vi "AlliGator Load Single Gate Image from SS2 mat File.vi"(6 "Action":T1, 8 "error in (no error)":errorcluster, 10 "File Info":variant, 11 "Gate Index":i32) -> (0 "error out":errorcluster, 1 "Data 2":sgl[][](array[numeric]), 3 "Data 1":sgl[][](array[numeric]))   [LabVIEW 2021, in "AlliGator Files.lvlib"]
doc: "Loads single gate image (or dual-channel images) from HDF5 FLI dataset file (v0.6b)."
uses:
  AlliGator Files.lvlib
  HDF5/AlliGator FLI Image Stack Action.ctl
  AlliGator SS2 mat FLI File Loading Information.ctl
  <vilib>/addons/h5labview2/file/H5F.lvlib
  GUI/AlliGator GUI.lvlib
  <vilib>/ErrorRing/Error Ring.xnode
  <vilib>/Utility/error.llb/Error Cluster From Error Code.vi
  <vilib>/addons/h5labview2/base/H5Equery.vi
  <vilib>/addons/h5labview2/base/lib_path.vi
  <vilib>/addons/h5labview2/dataset/H5Dread.llb/H5Dread.xnode
  HDF5/AlliGator HDF5.lvlib
panel:
  # "see the AlliGator License on the block diagram (Ctrl+E or Window:Show Block Diagram)"
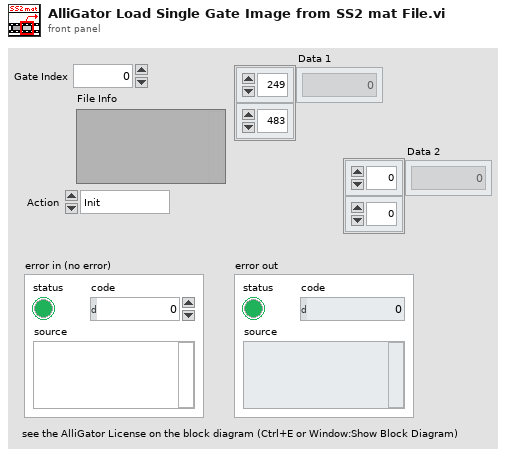
[diagram p1: front panel]
types:
  T1 = typedef "AlliGator HDF5.lvlib/AlliGator FLI Image Stack Action.ctl" = enum16{"Init", "Get Image", "Close"}
  T2 = typedef "AlliGator Files.lvlib/AlliGator SS2 mat FLI File Loading Information.ctl" = cluster{"mat File Path":path, "# Datasets":i32, "# Gates/Dataset":i32}
  T3 = typedef "hid_t.ctl" = i64
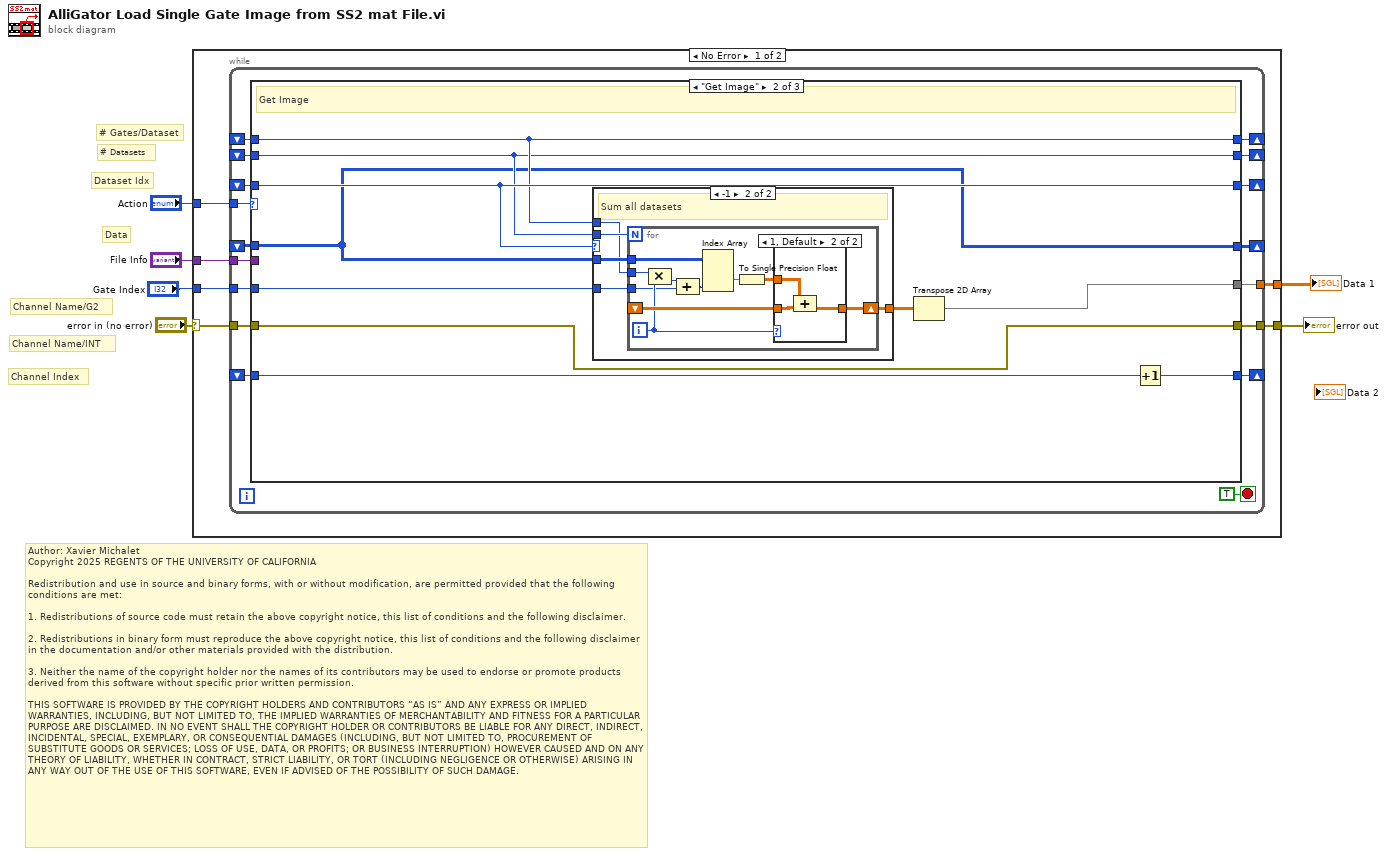
[diagram p0: block diagram]
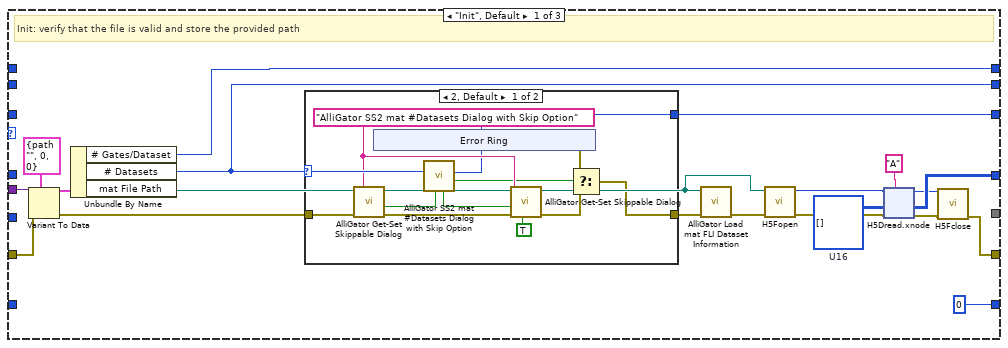
[diagram p2: hidden frame]
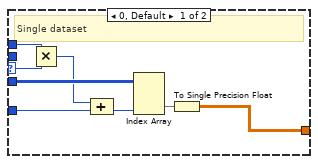
[diagram p4: hidden frame]
diagram:
  # "# Gates/Dataset"
  # "# Datasets"
  # "Dataset Idx"
  # "Data"
  # "Author: Xavier Michalet\nCopyright 2025 REGENTS OF THE UNIVERSITY OF CALIFORNIA\n\nRedistribution and use in source and binary forms, with or without modification, are permitted provided that the following conditions are met:\n\n1. Redistributions of source code must retain the above copyright notice, this list of conditions and the following disclaimer.\n\n2. Redistributions in binary form must reproduce the above copyright notice, this list of conditions and the following disclaimer in the documentation and/or other materials provided with the distribution.\n\n3. Neither the name of the copyright holder nor the names of its contributors may be used to endorse or promote products derived from this software without specific prior written permission.\n\nTHIS SOFTWARE IS PROVIDED BY THE COPYRIGHT HOLDERS AND CONTRIBUTORS “AS IS” AND ANY EXPRESS OR IMPLIED WARRANTIES, INCLUDING, BUT NOT LIMITED TO, THE IMPLIED WARRANTIES OF MERCHANTABILITY AND FITNESS FOR A PARTICULAR PURPOSE ARE DISCLAIMED. IN NO EVENT SHALL THE COPYRIGHT HOLDER OR CONTRIBUTORS BE LIABLE FOR ANY DIRECT, INDIRECT, INCIDENTAL, SPECIAL, EXEMPLARY, OR CONSEQUENTIAL DAMAGES (INCLUDING, BUT NOT LIMITED TO, PROCUREMENT OF SUBSTITUTE GOODS OR SERVICES; LOSS OF USE, DATA, OR PROFITS; OR BUSINESS INTERRUPTION) HOWEVER CAUSED AND ON ANY THEORY OF LIABILITY, WHETHER IN CONTRACT, STRICT LIABILITY, OR TORT (INCLUDING NEGLIGENCE OR OTHERWISE) ARISING IN ANY WAY OUT OF THE USE OF THIS SOFTWARE, EVEN IF ADVISED OF THE POSSIBILITY OF SUCH DAMAGE."
  # "Channel Index"
  # "Channel Name/INT"
  # "Channel Name/G2"
  n1 = case shown="No Error" "error in (no error)" {
    selector: "error in (no error)" -> [w11 w123]
    tunnel: [w10 w123] -> w5
    tunnel: "Action" -> [w12 _]
    tunnel: "File Info" -> [w9 _]
    tunnel: "Gate Index" -> [w8 _]
    tunnel: [w7 _] -> w1
    frame No Error {
      n2 = while {
        tunnel: w12 -> [w28]
        tunnel: w11 -> [w27]
        tunnel: [w26] -> w10
        tunnel: w9 -> [w25]
        tunnel: w8 -> [w24]
        tunnel: [w23] -> w7
        shift-right: [w22] -> _
        shift-left: _ -> [w21]
        shift-right: [w20] -> _
        shift-left: _ -> [w19]
        shift-right: [w18] -> _
        shift-left: _ -> [w16]
        shift-right: [w17] -> _
        shift-left: _ -> [w15]
        shift-right: [w14] -> _
        shift-left: _ -> [w13]
        stop <- TRUE stop-if-true
        n3 = case shown="\"Get Image\"" w28 {
          tunnel: w27 -> [w48 w82 w119]
          tunnel: [w30 w82 w119] -> w26
          tunnel: w25 -> [w49 _ _]
          tunnel: w24 -> [_ w87 _]
          tunnel: [_ w91 _] -> w23
          tunnel: w19 -> [_ w83 _]
          tunnel: [0 w89 _] -> w22
          tunnel: w21 -> [_ w90 _]
          tunnel: [w33 w83 _] -> w20
          tunnel: [w40 w86 w121] -> w18
          tunnel: [w39 w84 w122] -> w17
          tunnel: w16 -> [_ w86 w121]
          tunnel: w15 -> [_ w84 w122]
          tunnel: [w38 w85 w120] -> w14
          tunnel: w13 -> [_ w85 w120]
          frame "Init", Default {
            w37 = u16[][][] []  # U16
            # "Init: verify that the file is valid and store the provided path"
            n4 = Variant To Data(error in=w48, type=T2 {"mat File Path"=path "", "# Datasets"=0, "# Gates/Dataset"=0} ("SS2 mat File Loading Information"), Variant=w49) -> (data=w46:T2, error out=w42:errorcluster)
            n5 = Unbundle By Name(w46) -> ("# Gates/Dataset"=w38:i32, "# Datasets"=w39:i32, "mat File Path"=w43:path)
            n6 = case shown="2, Default" w39 {
              selector: w39 -> [w74 _]
              tunnel: w42 -> [w76 w81]
              tunnel: [w65 w81] -> w41
              tunnel: [w69 _] -> w40
              frame 2, Default {
                w72 = "AlliGator SS2 mat #Datasets Dialog with Skip Option" ("Dialog Window VI Name")
                n7 = call "AlliGator Get-Set Skippable Dialog.vi"("Error In"=w76, "Dialog Window VI Name"=w72) -> ("Error Out"=w73:errorcluster, "Is skipped (out)"=w75:bool)  [unwired: 8 in]
                n8 = xnode "Error Ring"() -> ("error out"=w66:errorcluster)
                n9 = call "AlliGator SS2 mat #Datasets Dialog with Skip Option.vi"("Do not show this dialog again"=w75, "# Repetitions"=w74) -> ("Cancel?"=w68:bool, "Dataset to Show (-1: all)"=w69:i32, "Do not show this dialog again?"=w71:bool)  [unwired: 6 in, 1 out]
                n10 = call "AlliGator Get-Set Skippable Dialog.vi"("Set/Get (F)"=TRUE, "Error In"=w73, "Is skipped (in)"=w71, "Dialog Window VI Name"=w72) -> ("Error Out"=w67:errorcluster)  [unwired: 6 in, 1 out]
                n11 = Select(t=w66, s=w68, f=w67) -> (s? t:f=w65:errorcluster)
              }
              frame 0, 1 {
              }
            }
            n12 = call "AlliGator Load mat FLI Dataset Information.vi"("Error In"=w41, "File Path"=w43) -> ("error out"=w44:errorcluster)  [unwired: 6 in, 3 out]
            n13 = call <vilib>:"H5Fopen.vi"("error in (no error)"=w44, "path"=w43) -> ("error out"=w34:errorcluster, "ref out"=w35:T3)  [unwired: 8 in]
            n14 = xnode "H5Dread.xnode"("dataset name (this)"="A", "error in (no error)"=w34, "default"=w37, "ref in"=w35) -> ("error out"=w31:errorcluster, "data"=w33:u16[][][], "ref out"=w32:i64)  [unwired: 2 in, 1 out]
            n15 = call <vilib>:"H5Fclose.vi"("error in (no error)"=w31, "ref"=w32) -> ("error out"=w30:errorcluster)  [unwired: 9 in]
          }
          frame "Get Image" {
            # "Get Image"
            n16 = case shown="-1" w86 {
              selector: w86 -> [w94 _]
              tunnel: [w99 w103] -> w88
              tunnel: w83 -> [w98 w102]
              tunnel: w87 -> [w97 w100]
              tunnel: w85 -> [w95 w101]
              tunnel: w84 -> [_ w104]
              frame 0, Default {
                # "Single dataset"
                n17 = Multiply(x=w95, y=w94) -> (x*y=w92:i32)
                n18 = Compound Arithmetic op=ADD(w92, w97) -> (w93:i32)
                n19 = Index Array(array=w98, index (dim 2)=w93) -> (element=w96:u16[][])  [unwired: 2 in]
                n20 = To Single Precision Float(number=w96) -> (single precision float=w99:sgl[][])
              }
              frame -1 {
                # "Sum all datasets"
                n21 = for {
                  N: w104 -> [_]
                  shift-right: [w113] -> w103
                  shift-left: _ -> [w110]
                  tunnel: w102 -> [w114]
                  tunnel: w101 -> [w109]
                  tunnel: w100 -> [w106]
                  i -> [w108]
                  n22 = Compound Arithmetic op=MULTIPLY(w109, w108) -> (w107:i32)
                  n23 = Compound Arithmetic op=ADD(w107, w106) -> (w105:i32)
                  n24 = Index Array(array=w114, index (dim 2)=w105) -> (element=w112:u16[][])  [unwired: 2 in]
                  n25 = To Single Precision Float(number=w112) -> (single precision float=w111:sgl[][])
                  n26 = case shown="1, Default" w108 {
                    tunnel: [w115 w116] -> w113
                    tunnel: w111 -> [w115 w117]
                    tunnel: w110 -> [_ w118]
                    frame 0 {
                    }
                    frame 1, Default {
                      n27 = Compound Arithmetic op=ADD(w117, w118) -> (w116:sgl[][])
                    }
                  }
                }
              }
            }
            n28 = Transpose 2D Array(2D array=w88) -> (transposed array=w91:sgl[][])
            n29 = Increment(x=w90) -> (x+1=w89:i32)
          }
          frame "Close" {
            # "Close File"
          }
        }
      }
    }
    frame Error {
    }
  }
  "Data 1" <- w1
  "error out" <- w5
